vi "Digital Trigger Detect (1 sample).vi"(11 "Digital Line Read":bool) -> (2 "Rising Edge":bool, 3 "Digital Line Read":bool)   [LabVIEW 2011]
doc: "This VI Detects rising edge on a specific digital line.\n\n<b> Latency = 0 Ticks <\\b>"
uses:
  <instrlib>/FlexRIO/Libraries/Helper VIs/NI FlexRIO Helper VIs.lvlib
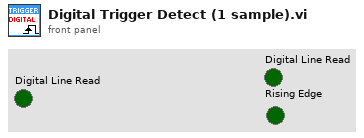
[diagram p1: front panel]
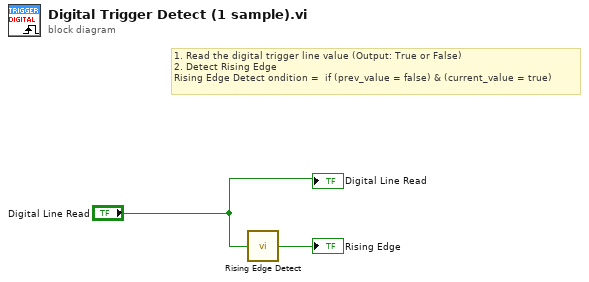
[diagram p0: block diagram]
diagram:
  # "1. Read the digital trigger line value (Output: True or False)\n2. Detect Rising Edge \nRising Edge Detect ondition =  if (prev_value = false) & (current_value = true)"
  n1 = call <instrlib>:"Rising Edge Detect.vi"("signal"="Digital Line Read") -> ("edge detected"=→"Rising Edge":bool)  [unwired: 14 in]
  "Digital Line Read" <- "Digital Line Read"
